vi "SV TDMS Write Waveform (N Ch).vi"(0 "tdms file":refnum<k34>, 1 "write channel properties (T)":bool=TRUE, 5 "group name in":string="Waveforms", 7 "channel names in":string[](array[string]), 9 "scaled signals":waveform(dbl)[](array[waveform]), 11 "error in":errorcluster) -> (4 "tdms file out":refnum<k34>, 6 "group name out":string, 8 "channel names out":string[](array[string]), 15 "error out":errorcluster)   [LabVIEW 2017]
doc: "Writes data to the specified .tdms file in a format specific to the polymorphic instance. Wire data to the <B>scaled signal [EU]</B> input to determine the polymorphic instance to use or manually select the instance."
uses:
  <vilib>/addons/_NISVFA/_Shared subVIs/Controls/LV Datatypes.ctl
  <vilib>/addons/_NISVFA/_Shared subVIs/Controls/NI Function Type.ctl
  <vilib>/addons/_NISVFA/_Shared subVIs/Controls/NI Function SubType.ctl
  <vilib>/addons/_NISVFA/_Shared subVIs/Controls/svc_X-Axis Units.ctl
  <vilib>/addons/_NISVFA/_Shared subVIs/Controls/svc_Unit Info.ctl
  <vilib>/addons/_NISVFA/_Shared subVIs/Common/svc_Engineering Units to Unit Label.vi
  <vilib>/addons/_NISVFA/_Shared subVIs/Common/svc_Unit Label to Engineering Units.vi
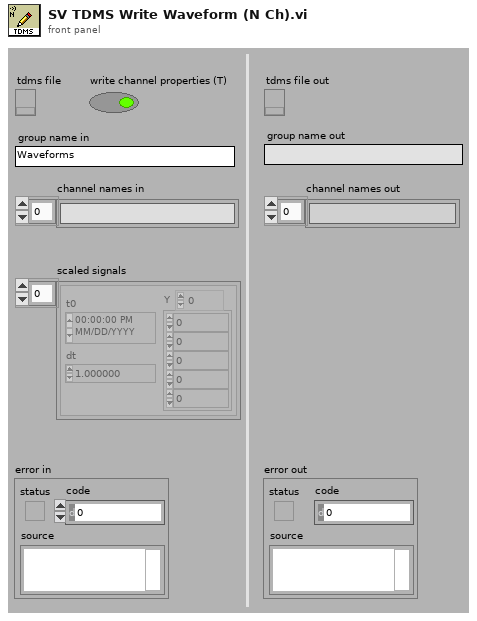
[diagram p1: front panel]
types:
  T1 = typedef "NI Function Type.ctl" = u16
  T2 = typedef "NI Function SubType.ctl" = u16
  T3 = typedef "svc_X-Axis Units.ctl" = u16
  T4 = cluster{"function type":T1, "function subtype":T2, "X-dimension":T3}
  T5 = typedef "LV Datatypes.ctl" = i32
  T6 = typedef "svc_Unit Info.ctl" = cluster{"X-axis label":string, "X-unit string":string, "Y-axis label":string, "Y-unit string":string}
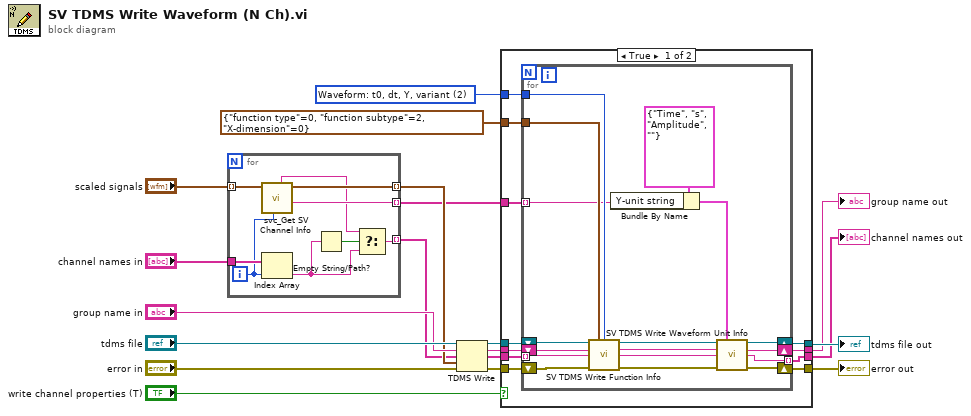
[diagram p0: block diagram]
diagram:
  w1 = T5 2 items=["String: abc"=-2, "Boolean: True or False"=-1, "Scalar: y"=0, "Array: Y"=1, "Waveform: t0, dt, Y, variant"=2, "Cluster: x0, dx, Y"=3, "Cluster: X, Y"=4, "Waterfall"=5, "Colormap"=6] ("LabVIEW datatype")
  n1 = for {
    tunnel: "scaled signals" -> [w28] mode=indexing
    tunnel: [w27] -> w6 mode=indexing
    tunnel: [w26] -> w5 mode=indexing
    tunnel: "channel names in" -> [w24]
    tunnel: [w22] -> w3 mode=indexing
    i -> [w23]
    n2 = call <vilib>:"svc_Get SV Channel Info.vi"("channel index"=w23, "scaled signal [EU]"=w28) -> ("unit label"=w26:string, "dup scaled signal [EU]"=w27:waveform(dbl), "channel name"=w25:string)  [unwired: 4 in, 3 out]
    n3 = Index Array(array=w24, index=w23) -> (element=w20:string)
    n4 = Empty String/Path?(string/path=w20) -> (empty?=w21:bool)
    n5 = Select(t=w25, s=w21, f=w20) -> (s? t:f=w22:string)
  }
  n6 = TDMS Write(0:"tdms file", 5:"group name in", 7:w3, 9:w6, 11:"error in") -> (4:w14:refnum<k34>, 6:w12:string, 8:w11:string[], 15:w9:errorcluster)  [unwired: 1 in]
  n7 = case shown="True" "write channel properties (T)" {
    tunnel: [w39 w60] -> w19
    tunnel: [w38 w59] -> w18
    tunnel: w9 -> [w37 w59]
    tunnel: w14 -> [w36 w60]
    tunnel: [w30 w58] -> w17
    tunnel: [w29 w57] -> w16
    tunnel: w12 -> [w35 w58]
    tunnel: w11 -> [w34 w57]
    tunnel: w5 -> [w33 _]
    tunnel: T4 {"function type"=0, "function subtype"=2, "X-dimension"=0} ("function info") -> [w32 _]
    tunnel: w1 -> [w31 _]
    frame True {
      n8 = for {
        shift-right: [w45] -> w39
        shift-left: w36 -> [w46]
        shift-right: [w50] -> w38
        shift-left: w37 -> [w49]
        tunnel: w34 -> [w48] mode=indexing
        tunnel: w33 -> [w41] mode=indexing
        tunnel: w32 -> [w56]
        tunnel: w31 -> [w55]
        tunnel: [w43] -> w29 mode=indexing
        shift-right: [w44] -> w30
        shift-left: w35 -> [w47]
        n9 = call <vilib>:"SV TDMS Write Function Info.vi"("tdms file in"=w46, "function info"=w56, "LabVIEW datatype"=w55, "group name"=w47, "channel name"=w48, "error in (no error)"=w49) -> ("tdms file out"=w54:refnum<k34>, "group name out"=w53:string, "channel name out"=w52:string, "error out"=w51:errorcluster)  [unwired: 6 in]
        n10 = Bundle By Name(cluster=T6 {"X-axis label"="Time", "X-unit string"="s", "Y-axis label"="Amplitude", "Y-unit string"=""} ("unit info"), "Y-unit string"=w41) -> (w40:T6)
        n11 = call <vilib>:"SV TDMS Write Waveform Unit Info.vi"("tdms file"=w54, "unit info"=w40, "group name"=w53, "channel name"=w52, "error in (no error)"=w51) -> ("tdms file out"=w45:refnum<k34>, "group name out"=w44:string, "channel name out"=w43:string, "error out"=w50:errorcluster)  [unwired: 7 in]
      }
    }
    frame False {
    }
  }
  "tdms file out" <- w19
  "error out" <- w18
  "channel names out" <- w16
  "group name out" <- w17
